vi "Decrement Counter.vi"(8 "error in (no error)":errorcluster, 11 "State Machine in":refnum<class "CCS_State Machine.lvclass">) -> (0 "error out":errorcluster, 2 "counter = zero":bool, 3 "State Machine out":refnum<class "CCS_State Machine.lvclass">)   [LabVIEW 2018, in "CCS_State Machine.lvclass"]
doc: "Decremet the counter of the class"
uses:
  CCS_State Machine.lvclass
  CCS_State Machine.lvclass/CCS_State Machine.ctl
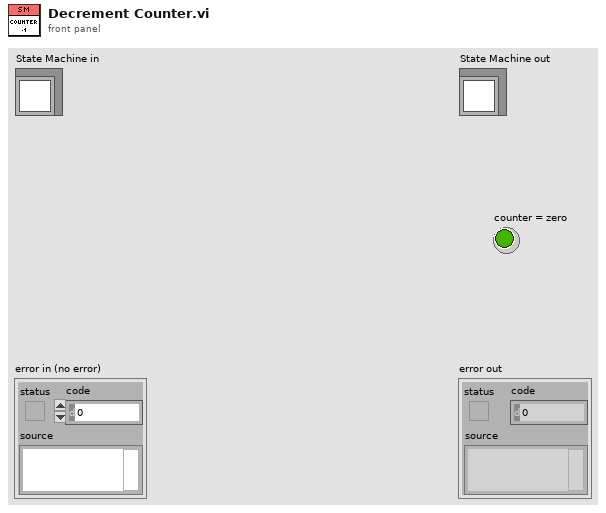
[diagram p1: front panel]
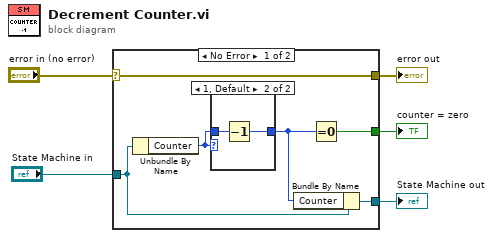
[diagram p0: block diagram]
diagram:
  n1 = case shown="No Error" "error in (no error)" {
    selector: "error in (no error)" -> [w11 w16]
    tunnel: [w11 w16] -> w4
    tunnel: [w9 w15] -> w2
    tunnel: "State Machine in" -> [w10 w15]
    tunnel: [w8 _] -> w1
    frame No Error {
      n2 = Unbundle By Name(w10) -> ("Counter"=w7:u16)
      n3 = case shown="1, Default" w7 {
        tunnel: w7 -> [w12 w14]
        tunnel: [w12 w13] -> w6
        frame 0 {
        }
        frame 1, Default {
          n4 = Decrement(x=w14) -> (x-1=w13:u16)
        }
      }
      n5 = Bundle By Name(cluster=w10, "Counter"=w6) -> (w9:refnum<class "CCS_State Machine.lvclass">)
      n6 = Equal To 0?(x=w6) -> (x = 0?=w8:bool)
    }
    frame Error {
    }
  }
  "error out" <- w4
  "State Machine out" <- w2
  "counter = zero" <- w1
